vi "Get value string.vi"(8 "error in (no error)":errorcluster, 11 "Column in":refnum<class "Ctrl Refnum Column.lvclass">) -> (0 "error out":errorcluster, 2 "Value":string, 3 "Column out":refnum<class "Ctrl Refnum Column.lvclass">)   [LabVIEW 2020, in "Basic Fields.lvlib" / "Ctrl Refnum Column.lvclass"]
uses:
  Ctrl Refnum Column.lvclass
  Ctrl Refnum Column.lvclass/Ctrl Refnum Column.ctl
  Basic Columns/Basic Columns/Column Class/Column Parent.lvclass
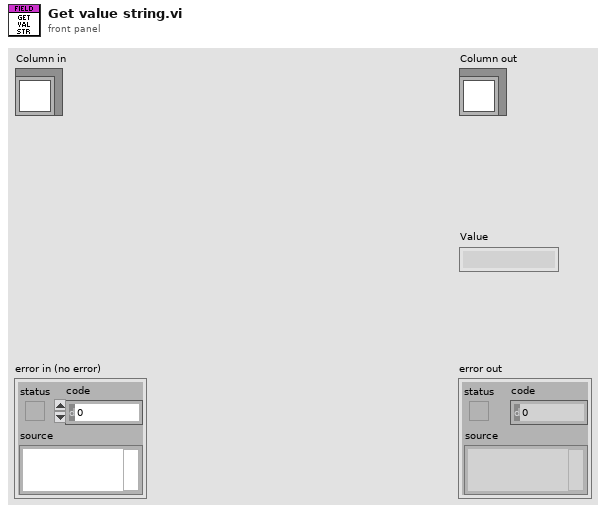
[diagram p1: front panel]
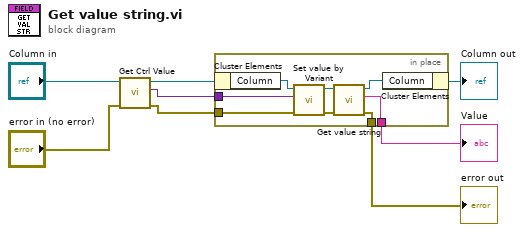
[diagram p0: block diagram]
diagram:
  n1 = call-dynamic "Get Ctrl Value.vi"("error in (no error)"="error in (no error)", "Ctrl Refnum Column in"="Column in") -> ("error out"=w2:errorcluster, "Ctrl Value"=w6:variant, "Ctrl Refnum Column out"=w7:refnum<class "Ctrl Refnum Column.lvclass">)  [unwired: 7 in]
  n2 = in-place {
    in-place-border: w6 -> [w13]
    in-place-border: [w11] -> w5
    in-place-border: w2 -> [w10]
    in-place-border: [w9] -> w1
    n3 = in-place-cluster #1(w7) -> ("Column"=w16:refnum<class "Column Parent.lvclass">)
    n4 = call-dynamic "Set value by Variant.vi"("error in (no error)"=w10, "Variant"=w13, "Column in"=w16) -> ("error out"=w12:errorcluster, "Column out"=w15:refnum<class "Column Parent.lvclass">)  [unwired: 7 in]
    n5 = call-dynamic "Get value string.vi"("error in (no error)"=w12, "Column in"=w15) -> ("error out"=w9:errorcluster, "Value"=w11:string, "Column out"=w14:refnum<class "Column Parent.lvclass">)  [unwired: 7 in]
    n6 = in-place-cluster #1("Column"=w14) -> (→"Column out":refnum<class "Ctrl Refnum Column.lvclass">)
  }
  "error out" <- w1
  "Value" <- w5
